vi "Shift.vi"(1 "LeftMotor1Ref":T1={"DeviceStatus"={"status"=FALSE, "code"=0, "source"=""}, "Type"=enum."PWM", "PWM"={"PWM Channel"=enum."PWM 1", "DeadBand"={"Name"="", "maxPositivePwm"=0, "minPositivePwm"=0, "centerPwm"=0, "maxNegativePwm"=0, "minNegativePwm"=0, "angularRange"=0}}, "CAN"={"Device Number"=0, "Control Mode"=enum."Percent VBus", "Semaphore"=refnum, "Max Vout"=12.0, "TalonSRX Control Mode"=enum."Percent VBus"}, "Invert"=FALSE}, 7 "Buttons":bool[](array[boolean]), 9 "CalculatedLeftMotorOutput":dbl, 11 "CalculatedRightMotorOutput":dbl, 12 "RightMotor1Ref":T1={"DeviceStatus"={"status"=FALSE, "code"=0, "source"=""}, "Type"=enum."PWM", "PWM"={"PWM Channel"=enum."PWM 1", "DeadBand"={"Name"="", "maxPositivePwm"=0, "minPositivePwm"=0, "centerPwm"=0, "maxNegativePwm"=0, "minNegativePwm"=0, "angularRange"=0}}, "CAN"={"Device Number"=0, "Control Mode"=enum."Percent VBus", "Semaphore"=refnum, "Max Vout"=12.0, "TalonSRX Control Mode"=enum."Percent VBus"}, "Invert"=FALSE}) -> (4 "LeftMotorOutput":dbl, 15 "RightMotorOutput":dbl)   [LabVIEW 2015]
uses:
  <vilib>/Rock Robotics/WPI/MotorControl/WPI_MotorControlDeviceRef.ctl
  <vilib>/Rock Robotics/WPI/MotorControl/WPI_MotorControlType.ctl
  <vilib>/Rock Robotics/SystemInterfaces/DIO/FPGA_DIOPWMChannel.ctl
  <vilib>/Rock Robotics/WPI/PWM/WPI_PWMDeadband.ctl
  <vilib>/Rock Robotics/WPI/CAN/Jaguar/SubVIs/WPI_CANJaguar_ControlMode.ctl
  <vilib>/Rock Robotics/WPI/CAN/TalonSRX/WPI_CANTalonSRX_APIControlMode.ctl
  Utilities/ShiftControl.ctl
  Utilities/ShiftGlobals.vi
  Utilities/GlobalButtons.vi
panel:
  out "Shifting":bool
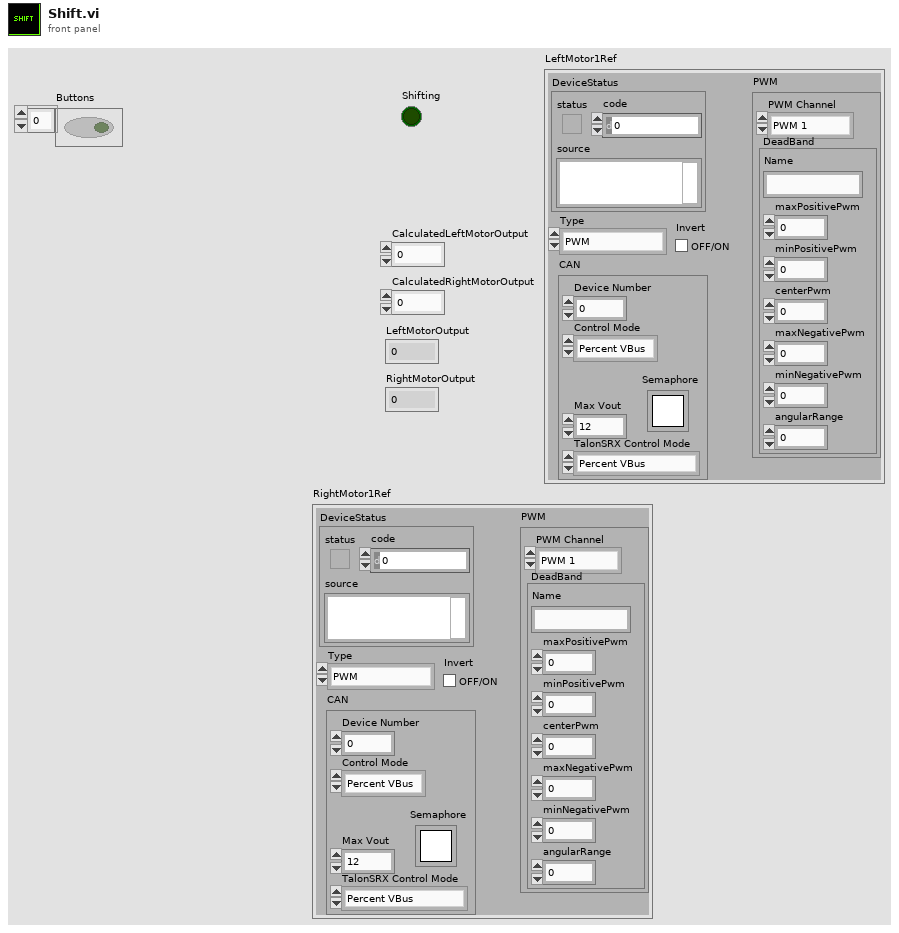
[diagram p1: front panel]
types:
  T1 = typedef "WPI_MotorControlDeviceRef.ctl" = cluster{"DeviceStatus":errorcluster, "Type":T2, "PWM":cluster{"PWM Channel":T3, "DeadBand":T4}, "CAN":cluster{"Device Number":u8, "Control Mode":T5, "Semaphore":T6, "Max Vout":dbl, "TalonSRX Control Mode":T7}, "Invert":bool}
  T2 = typedef "WPI_MotorControlType.ctl" = enum16{"PWM", "CAN", "CANTalonSRX"}
  T3 = typedef "FPGA_DIOPWMChannel.ctl" = enum8{"PWM 0", "PWM 1", "PWM 2", "PWM 3", "PWM 4", "PWM 5", "PWM 6", "PWM 7", "PWM 8", "PWM 9", "PWM MXP 0", "PWM MXP 1", "PWM MXP 2", "PWM MXP 3", "PWM MXP 4", "PWM MXP 5", "PWM MXP 6", "PWM MXP 7", "PWM MXP 8", "PWM MXP 9", "Invalid"}
  T4 = typedef "WPI_PWMDeadband.ctl" = cluster{"Name":string, "maxPositivePwm":i32, "minPositivePwm":i32, "centerPwm":i32, "maxNegativePwm":i32, "minNegativePwm":i32, "angularRange":u16}
  T5 = typedef "WPI_CANJaguar_ControlMode.ctl" = enum8{"Percent VBus", "Current", "Speed", "Position", "Voltage"}
  T6 = typedef "Semaphore RefNum" = refnum<k1>
  T7 = typedef "WPI_CANTalonSRX_APIControlMode.ctl" = enum8{"Percent VBus", "Speed", "Position", "Slave", "Unchanged / Invalid", "Voltage Compensation", "Current", "Motion Profile"}
  T8 = typedef "ShiftControl.ctl" = enum16{"WaitingForInput", "Shift", "CutPower", "ReEngagePower"}
  T9 = typedef "WPI_CANTalonSRX_GlobalStatus.ctl" = cluster{"Applied Throttle":dbl, "Module Enabled":bool, "CAN Error":errorcluster, "Closed Loop Error":dbl, "Forward Limit Switch Closed":bool, "Reverse Limit Switch Closed":bool, "Sensor Position":dbl, "Sensor Velocity":dbl, "Current":dbl, "Sticky Fault - Over Temp":bool, "Sticky Fault - Under Voltage":bool, "Sticky Fault - Forward Limit":bool, "Sticky Fault - Reverse Limit":bool, "Sticky Fault - Forward Soft Limit":bool, "Sticky Fault - Reverse Soft Limit":bool, "Brake is Enabled":bool, "Encoder Position":dbl, "Encoder Velocity":dbl, "Encoder Index Count":dbl, "Encoder A Pin State":bool, "Encoder B Pin State":bool, "Encoder Index Pin State":bool, "Analog In":dbl, "Analog In Velocity":dbl, "Temperature (C)":dbl, "Battery Voltage":dbl, "Control 5 Is Supported":bool, "Current Profile Slot Select":dbl, "Pos Div 8":bool, "Vel Div 4":bool, "Pulse Width Position":i32, "Pulse Width Velocity":i32, "Pulse Width Rise To Rise (us)":i32, "Pulse Width Rise To Fall (us)":i32, "Mot Prof Active Is Under Run":bool, "Mot Prof Active Has Under Run":bool, "Mot Prof Active Is Last":bool, "Mot Prof Active Velocity Only":bool, "Mot Prof Active Is Valid":bool, "Mot Prof Buffer Is Full":bool, "Mot Prof Active Profile Slot Select":i32, "Mot Prof NextID":i32, "Mot Prof Count":i32, "Mot Prof Active Velocity":dbl, "Mot Prof Active Position":dbl, "Mot Prof Output Enable":i32}
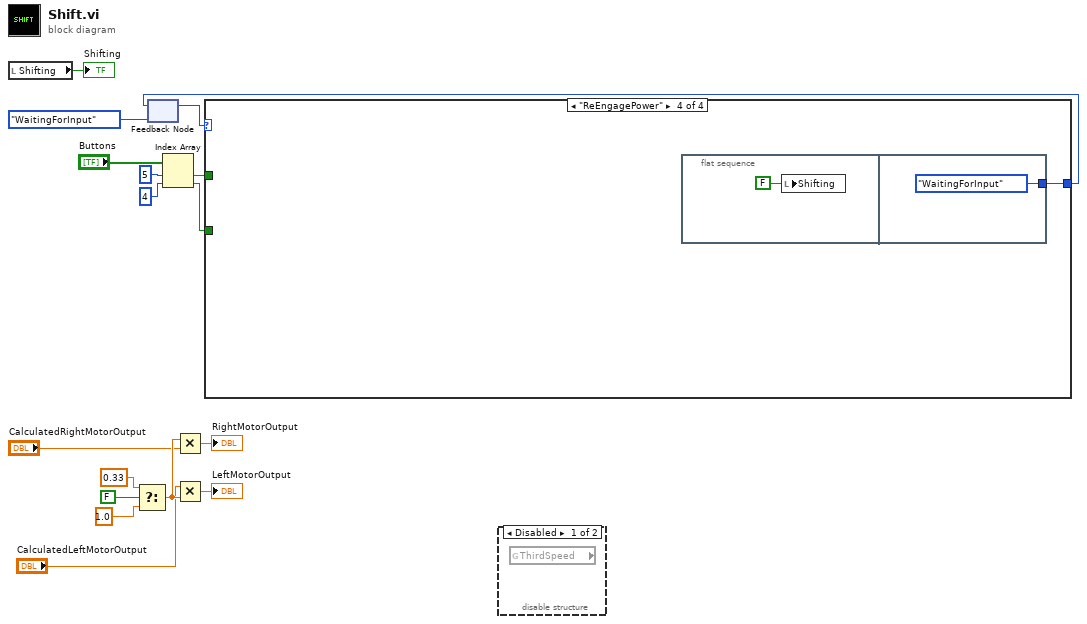
[diagram p0: block diagram]
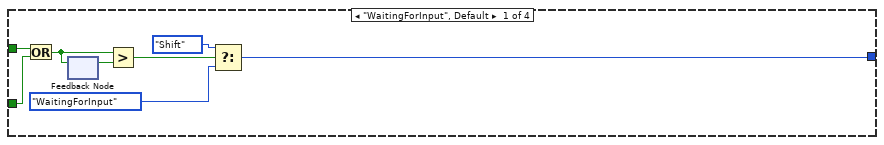
[diagram p3: hidden frame]
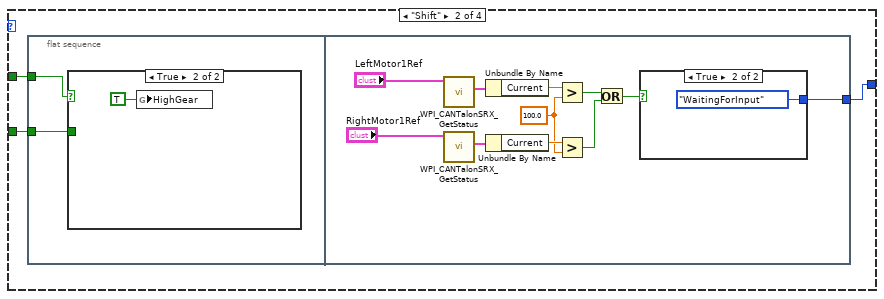
[diagram p4: hidden frame]
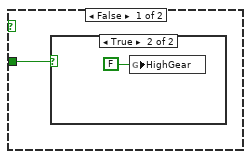
[diagram p5: hidden frame]
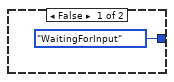
[diagram p7: hidden frame]
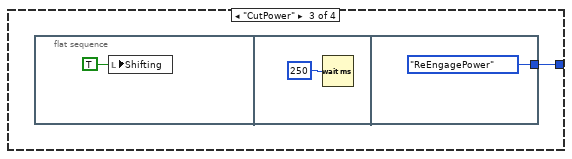
[diagram p8: hidden frame]
diagram:
  n1 = local read "Shifting"() -> (→"Shifting":bool)
  n2 = Select(t=0.33, s=FALSE, f=1.0) -> (s? t:f=w13:dbl)
  n3 = feedback #1(ShiftControl."WaitingForInput" ("Shift")) -> (w16:T8)
  n4 = Index Array(array="Buttons", index #1=5 ("index"), index #2=4 ("index")) -> (element #1=w3:bool, element #2=w4:bool)
  n5 = Multiply(x=w13, y="CalculatedRightMotorOutput") -> (x*y=→"RightMotorOutput":dbl)
  n6 = Multiply(x="CalculatedLeftMotorOutput", y=w13) -> (x*y=→"LeftMotorOutput":dbl)
  n7 = case shown="\"ReEngagePower\"" w16 {
    tunnel: [w23 w28 w47 w51] -> w15
    tunnel: w4 -> [w22 w26 _ _]
    tunnel: w3 -> [w21 w27 _ _]
    frame "WaitingForInput", Default {
      n8 = Or(x=w21, y=w22) -> (x .or. y?=w19:bool)
      n9 = feedback-in #2(w19) -> ()
      n10 = feedback #2() -> (w20:bool)  [unwired: 1 in]
      n11 = Greater?(x=w19, y=w20) -> (0:w18:bool)
      n12 = Select(t=ShiftControl."Shift" ("Shift"), s=w18, f=ShiftControl."WaitingForInput" ("Shift")) -> (s? t:f=w23:T8)
    }
    frame "Shift" {
      n13 = flat-sequence {
        tunnel: w27 -> [w30]
        tunnel: w26 -> [w29]
        tunnel: [w37] -> w28
        frame #0 {
          n14 = case shown="True" w30 {
            tunnel: w29 -> [w31 _]
            frame False {
              n15 = case shown="True" w31 {
                frame False {
                }
                frame True {
                  n16 = global write "ShiftGlobals.vi" "HighGear"(FALSE ("HighGear")) -> ()
                }
              }
            }
            frame True {
              n17 = global write "ShiftGlobals.vi" "HighGear"(TRUE ("HighGear")) -> ()
            }
          }
        }
        frame #1 {
          w38 = 100.0
          n18 = call <vilib>:"WPI_CANTalonSRX_GetStatus.vi"("CAN Talon SRX Ref"="LeftMotor1Ref") -> ("Talon SRX Status"=w41:T9)  [unwired: 8 in, 2 out]
          n19 = call <vilib>:"WPI_CANTalonSRX_GetStatus.vi"("CAN Talon SRX Ref"="RightMotor1Ref") -> ("Talon SRX Status"=w44:T9)  [unwired: 8 in, 2 out]
          n20 = Unbundle By Name(w41) -> ("Current"=w40:dbl)
          n21 = Unbundle By Name(w44) -> ("Current"=w39:dbl)
          n22 = Greater?(x=w40, y=w38) -> (0:w36:bool)
          n23 = Greater?(x=w39, y=w38) -> (0:w35:bool)
          n24 = Or(x=w36, y=w35) -> (x .or. y?=w34:bool)
          n25 = case shown="True" w34 {
            tunnel: [ShiftControl."WaitingForInput" ("Shift") ShiftControl."WaitingForInput" ("Shift")] -> w37
            frame False {
            }
            frame True {
            }
          }
        }
      }
    }
    frame "CutPower" {
      n26 = flat-sequence {
        tunnel: [ShiftControl."ReEngagePower" ("Shift")] -> w47
        frame #0 {
          n27 = local write "Shifting"(TRUE ("Shifting")) -> ()
        }
        frame #1 {
          n28 = Wait (ms)(milliseconds to wait=u32 250) -> ()  [unwired: 1 out]
        }
        frame #2 {
        }
      }
    }
    frame "ReEngagePower" {
      n29 = flat-sequence {
        tunnel: [ShiftControl."WaitingForInput" ("Shift")] -> w51
        frame #0 {
          n30 = local write "Shifting"(FALSE ("Shifting")) -> ()
        }
        frame #1 {
        }
      }
    }
  }
  n31 = feedback-in #1(w15) -> ()
  n32 = disable-structure shown="Disabled" {
    frame Disabled {
      n33 = global read "GlobalButtons.vi" "ThirdSpeed"() -> ()  [unwired: 1 out]
    }
    frame Enabled {
    }
  }
